vi "Update Device Status Listbox.vi"(9 "DeviceIDs":T1[](array[typedef]), 10 "queue in":refnum<queue>, 11 "EMS User Interface in":refnum<class "EMS User Interface.lvclass">) -> ()   [LabVIEW 2018, in "EMS User Interface Actor.lvlib" / "EMS User Interface.lvclass"]
uses:
  EMS User Interface.lvclass
  C:/Users/Administrator/Desktop/2018LabVIEW EMS/EMS Generic Actor/EMS Generic/EMS Generic.lvclass
  EMS Generic Actor/EMS Generic/Controls/Device Information Cluster.ctl
  EMS Generic Actor/EMS Generic/Controls/Device State.ctl
  <vilib>/ORNL/CSEISMIC DDS/CSEISMIC DDS Base/Data Types/Controls/DeviceID.ctl
  EMS Generic Actor/EMS Generic/EMS Generic.lvclass
  <vilib>/ORNL/CSEISMIC DDS/CSEISMIC DDS Base/CSEISMIC DDS.lvclass
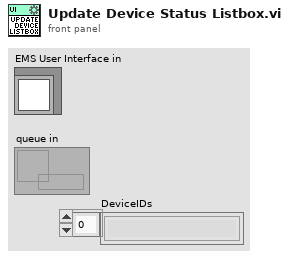
[diagram p1: front panel]
types:
  T1 = typedef "CSEISMIC DDS.lvlib/CSEISMIC DDS.lvclass/DeviceID.ctl" = string
  T2 = typedef "EMS Generic Actor.lvlib/EMS Generic.lvclass/Device Information Cluster.ctl" = cluster{"Device State":T3, "data":variant}
  T3 = typedef "EMS Generic Actor.lvlib/EMS Generic.lvclass/Device State.ctl" = enum16{"Invalid", "Clear", "DevIDs in Config", "DevIDs on uGrid", "DevIDs not on uGrid", "Update IED_Status", "Update DER_Status", "Update DER_Measurement", "Update SmartRelay_Measurement"}
  T4 = typedef "CSEISMIC DDS.lvlib/CSEISMIC DDS.lvclass/IED_Status.ctl" = cluster{"DeviceID":T1, "Timestamp":T5, "MicrogridID":u8, "Active":bool, "Inactive":bool, "Error":i32, "Fault":bool, "ErrorString":string}
  T5 = typedef "CSEISMIC DDS.lvlib/CSEISMIC DDS.lvclass/Timestamp.ctl" = cluster{"Seconds":u64, "Remainder":u64}
  T6 = typedef "CSEISMIC DDS.lvlib/CSEISMIC DDS.lvclass/DER_Status.ctl" = cluster{"DeviceID":T1, "VFControl":bool, "PControl":bool, "QControl":bool, "PFControl":bool, "PVControl":bool, "Droop":bool, "Unbalanced":bool, "MicrogridVF":bool, "RealDroop(kW)":T7, "ReactiveDroop(kVar)":T7}
  T7 = typedef "CSEISMIC DDS.lvlib/CSEISMIC DDS.lvclass/DroopCurve.ctl" = cluster{"XMin":dbl, "XMax":dbl, "YMin":dbl, "YMax":dbl}
  T8 = typedef "CSEISMIC DDS.lvlib/CSEISMIC DDS.lvclass/DER_Measurement.ctl" = cluster{"DeviceID":T1, "Voltage":dbl[], "Current":dbl[], "RealPower":dbl[], "ReactivePower":dbl[], "LineConfig":u8[], "Frequency":dbl}
  T9 = typedef "CSEISMIC DDS.lvlib/CSEISMIC DDS.lvclass/SmartRelay_Measurement.ctl" = cluster{"DeviceID":T1, "PrimaryVoltage":dbl[], "SecondaryVoltage":dbl[], "Current":dbl[], "RealPower":dbl[], "ReactivePower":dbl[], "LineConfig":u8[], "Frequency":dbl}
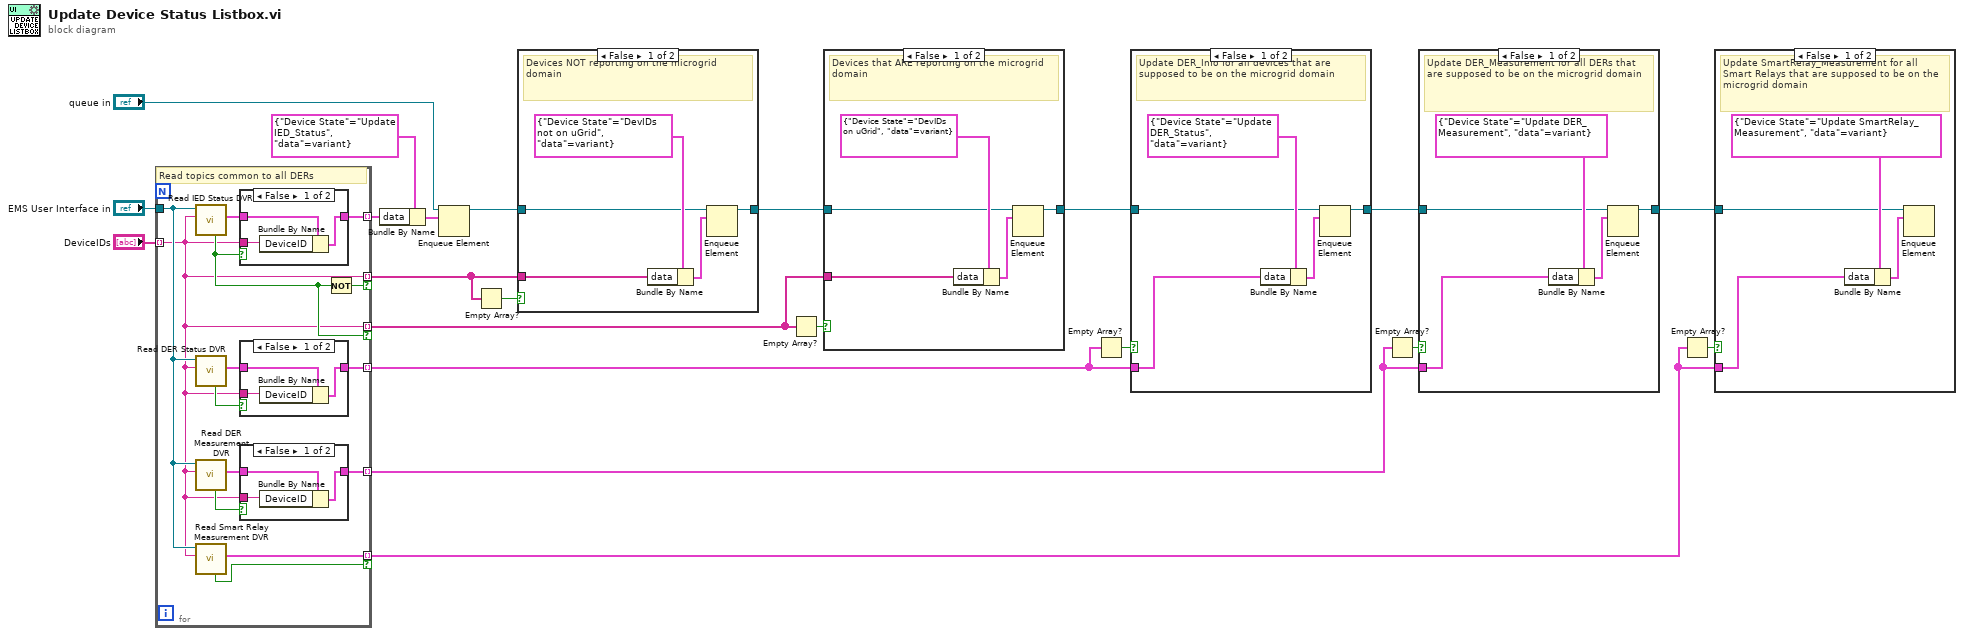
[diagram p0: block diagram]
diagram:
  n1 = for {
    tunnel: "EMS User Interface in" -> [w25]
    tunnel: "DeviceIDs" -> [w22] mode=indexing
    tunnel: [w33] -> w17 mode=indexing
    tunnel: [w22] -> w14 mode=indexing if=w35
    tunnel: [w22] -> w12 mode=indexing if=w32
    tunnel: [w30] -> w8 mode=indexing
    tunnel: [w26] -> w5 mode=indexing
    tunnel: [w24] -> w2 mode=indexing if=w23
    # "Read topics common to all DERs"
    n2 = call "Read IED Status DVR.vi"("DeviceID"=w22, "EMS Generic in"=w25) -> ("IED_Status"=w34:T4, "valid?"=w32:bool)  [unwired: 6 in, 2 out]
    n3 = call "Read DER Status DVR.vi"("DeviceID"=w22, "EMS Generic in"=w25) -> ("DER_Status"=w31:T6, "valid?"=w29:bool)  [unwired: 6 in, 2 out]
    n4 = call "Read DER Measurement DVR.vi"("DeviceID"=w22, "EMS Generic in"=w25) -> ("DER_Measurement"=w27:T8, "valid?"=w28:bool)  [unwired: 6 in, 2 out]
    n5 = call "Read Smart Relay Measurement DVR.vi"("DeviceID"=w22, "EMS Generic in"=w25) -> ("SmartRelay_Measurement"=w24:T9, "valid?"=w23:bool)  [unwired: 6 in, 2 out]
    n6 = case shown="False" w32 {
      tunnel: w34 -> [w46 w47]
      tunnel: [w45 w47] -> w33
      tunnel: w22 -> [w44 _]
      frame False {
        n7 = Bundle By Name(cluster=w46, "DeviceID"=w44) -> (w45:T4)
      }
      frame True {
      }
    }
    n8 = case shown="False" w29 {
      tunnel: w31 -> [w42 w43]
      tunnel: [w41 w43] -> w30
      tunnel: w22 -> [w40 _]
      frame False {
        n9 = Bundle By Name(cluster=w42, "DeviceID"=w40) -> (w41:T6)
      }
      frame True {
      }
    }
    n10 = case shown="False" w28 {
      tunnel: w27 -> [w38 w39]
      tunnel: [w37 w39] -> w26
      tunnel: w22 -> [w36 _]
      frame False {
        n11 = Bundle By Name(cluster=w38, "DeviceID"=w36) -> (w37:T8)
      }
      frame True {
      }
    }
    n12 = Not(x=w32) -> (.not. x?=w35:bool)
  }
  n13 = Bundle By Name(cluster=T2 {"Device State"=enum."Update IED_Status", "data"=variant} ("Device State Information"), "data"=w17) -> (w16:T2)
  n14 = Enqueue Element(queue="queue in", element=w16) -> (queue out=w15:refnum<queue>)  [unwired: 2 in, 2 out]
  n15 = Empty Array?(array=w14) -> (empty?=w13:bool)
  n16 = case shown="False" w13 {
    tunnel: w14 -> [w51 _]
    tunnel: w15 -> [w49 w53]
    tunnel: [w48 w53] -> w10
    frame False {
      # "Devices NOT reporting on the microgrid domain"
      n17 = Bundle By Name(cluster=T2 {"Device State"=enum."DevIDs not on uGrid", "data"=variant} ("Device State Information"), "data"=w51) -> (w52:T2)
      n18 = Enqueue Element(queue=w49, element=w52) -> (queue out=w48:refnum<queue>)  [unwired: 2 in, 2 out]
    }
    frame True {
      # "All devices are reporting on the microgrid domain"
    }
  }
  n19 = Empty Array?(array=w12) -> (empty?=w11:bool)
  n20 = case shown="False" w11 {
    tunnel: w12 -> [w57 _]
    tunnel: w10 -> [w55 w59]
    tunnel: [w54 w59] -> w9
    frame False {
      # "Devices that ARE reporting on the microgrid domain"
      n21 = Bundle By Name(cluster=T2 {"Device State"=enum."DevIDs on uGrid", "data"=variant} ("Device State Information"), "data"=w57) -> (w58:T2)
      n22 = Enqueue Element(queue=w55, element=w58) -> (queue out=w54:refnum<queue>)  [unwired: 2 in, 2 out]
    }
    frame True {
      # "No devices are reporting on the microgrid domain"
    }
  }
  n23 = Empty Array?(array=w8) -> (empty?=w7:bool)
  n24 = case shown="False" w7 {
    tunnel: w9 -> [w62 w65]
    tunnel: w8 -> [w61 _]
    tunnel: [w60 w65] -> w6
    frame False {
      # "Update DER_Info for all devices that are supposed to be on the microgrid domain"
      n25 = Bundle By Name(cluster=T2 {"Device State"=enum."Update DER_Status", "data"=variant} ("Device State Information"), "data"=w61) -> (w64:T2)
      n26 = Enqueue Element(queue=w62, element=w64) -> (queue out=w60:refnum<queue>)  [unwired: 2 in, 2 out]
    }
    frame True {
      # "No devices are reporting on the microgrid domain"
    }
  }
  n27 = Empty Array?(array=w5) -> (empty?=w4:bool)
  n28 = case shown="False" w4 {
    tunnel: w6 -> [w68 w71]
    tunnel: w5 -> [w67 _]
    tunnel: [w66 w71] -> w3
    frame False {
      # "Update DER_Measurement for all DERs that are supposed to be on the microgrid domain"
      n29 = Bundle By Name(cluster=T2 {"Device State"=enum."Update DER_Measurement", "data"=variant} ("Device State Information"), "data"=w67) -> (w70:T2)
      n30 = Enqueue Element(queue=w68, element=w70) -> (queue out=w66:refnum<queue>)  [unwired: 2 in, 2 out]
    }
    frame True {
      # "No DERs are reporting on the microgrid domain"
    }
  }
  n31 = Empty Array?(array=w2) -> (empty?=w1:bool)
  n32 = case shown="False" w1 {
    tunnel: w3 -> [w73 _]
    tunnel: w2 -> [w72 _]
    frame False {
      # "Update SmartRelay_Measurement for all Smart Relays that are supposed to be on the microgrid domain"
      n33 = Bundle By Name(cluster=T2 {"Device State"=enum."Update SmartRelay_Measurement", "data"=variant} ("Device State Information"), "data"=w72) -> (w75:T2)
      n34 = Enqueue Element(queue=w73, element=w75) -> ()  [unwired: 2 in, 3 out]
    }
    frame True {
      # "No Smart Relays are reporting on the microgrid domain"
    }
  }
